vi "QPSK.vi"() -> ()   [LabVIEW 2018]
uses:
  <vilib>/addons/Modulation/Digital/General/MT Generate Bits (Galois, PN Order).vi
  <vilib>/addons/Modulation/Digital/Support/Common/Validators/mod_Generate Bits Validate.vi
  <vilib>/addons/Modulation/Analog/support/mod_Set Error Source.vi
  <vilib>/addons/Modulation/Digital/General/subVIs/mod_Generate Bits PN Sequence.vi
  <vilib>/addons/Modulation/niDMT.lvlib
  <vilib>/Analysis/NI_AALBase.lvlib
panel:
  out "Gaussian noise pattern":dbl[](array[numeric])
  out "X * Y":cdb[](array[numeric])
  out "output of Bpsk mapper":cdb[](array[numeric])
  out "x+y":cdb[](array[numeric])
  in  "samples":i32=128
  in  "pulse shaping samples per symbol (16)":i32
  in  "modulation type":T1(ring)
  in  "pulse shaping filter (none)":T2(ring)
  in  "PN sequence order (9)":i32=9
  in  "total bits (128)":i32=128
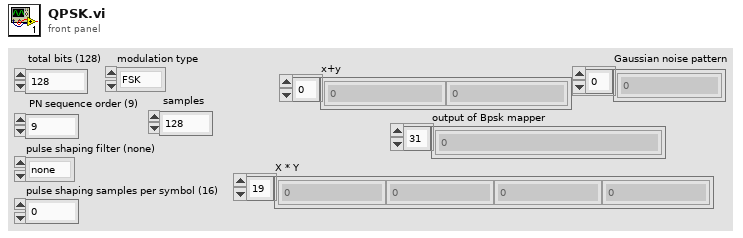
[diagram p1: front panel]
types:
  T1 = enum16{"FSK", "PSK", "QAM", "MSK", "PAM", "ASK", "CPM"}
  T2 = enum16{"none", "Raised Cosine", "Root Raised Cos", "Gaussian"}
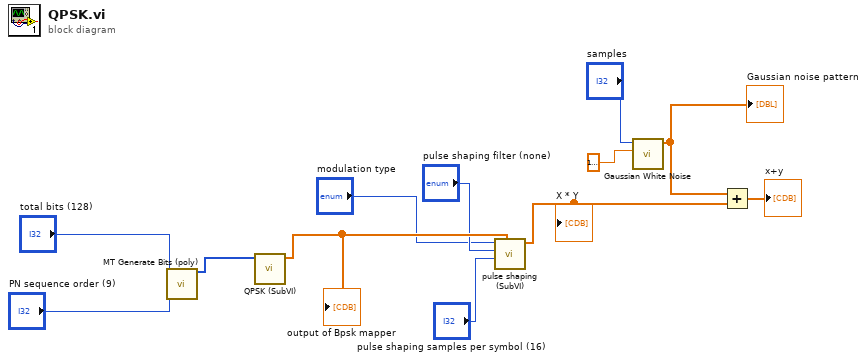
[diagram p0: block diagram]
diagram:
  n1 = call-poly <vilib>:"MT Generate Bits (poly).vi"("total bits (128)"="total bits (128)", "PN sequence order (9)"="PN sequence order (9)") -> ("output bit stream"=w12:i8[])  [unwired: 11 in, 2 out]
  n2 = call "QPSK (SubVI).vi"("output bit stream"=w12) -> ("Array"=w9:cdb[])  [unwired: 10 in]
  "output of Bpsk mapper" <- w9
  n3 = call "pulse shaping (SubVI).vi"("IQ symbols"=w9, "pulse shaping samples per symbol (16)"="pulse shaping samples per symbol (16)", "pulse shaping filter (none)"="pulse shaping filter (none)", "modulation type"="modulation type") -> ("X * Y"=w4:cdb[])  [unwired: 7 in]
  "X * Y" <- w4
  n4 = call <vilib>:"Gaussian White Noise.vi"("standard deviation"=1.0000000000000002, "samples"="samples") -> ("Gaussian noise pattern"=w5:dbl[])  [unwired: 8 in, 1 out]
  "Gaussian noise pattern" <- w5
  n5 = Add(x=w5, y=w4) -> (x+y=→"x+y":cdb[])
